vi "Parse Module Specifications.vi"(11 "Module Spec. File":path) -> (0 "Type Categories":T1, 1 "Namespaces":T12[](array[typedef]), 2 "Projections":T13[](array[typedef]), 3 "Module Name":string)   [LabVIEW 2013]
uses:
  Data Structures/JSON/Projection Info.ctl
  Data Structures/JSON/Namespace.ctl
  Data Structures/JSON/Enum.ctl
  Data Structures/JSON/Enum Value.ctl
  Data Structures/JSON/Method.ctl
  Data Structures/JSON/Param.ctl
  Data Structures/JSON/Connector Pane.ctl
  Data Structures/JSON/Connector Pane Terminal.ctl
  Data Structures/JSON/Type Categories.ctl
  Data Structures/JSON/TypeConv.ctl
  Data Structures/JSON/Simple Struct.ctl
  Data Structures/JSON/Class.ctl
  Data Structures/JSON/Property.ctl
  <vilib>/addons/JSON API/JSON Object/JSON Object.lvclass
  <vilib>/addons/JSON API/JSON Value/JSON Value.lvclass
  <vilib>/addons/JSON API/JSON Scalar/JSON Scalar.lvclass
  <vilib>/addons/JSON API/Variant JSON/Variant JSON.lvlib
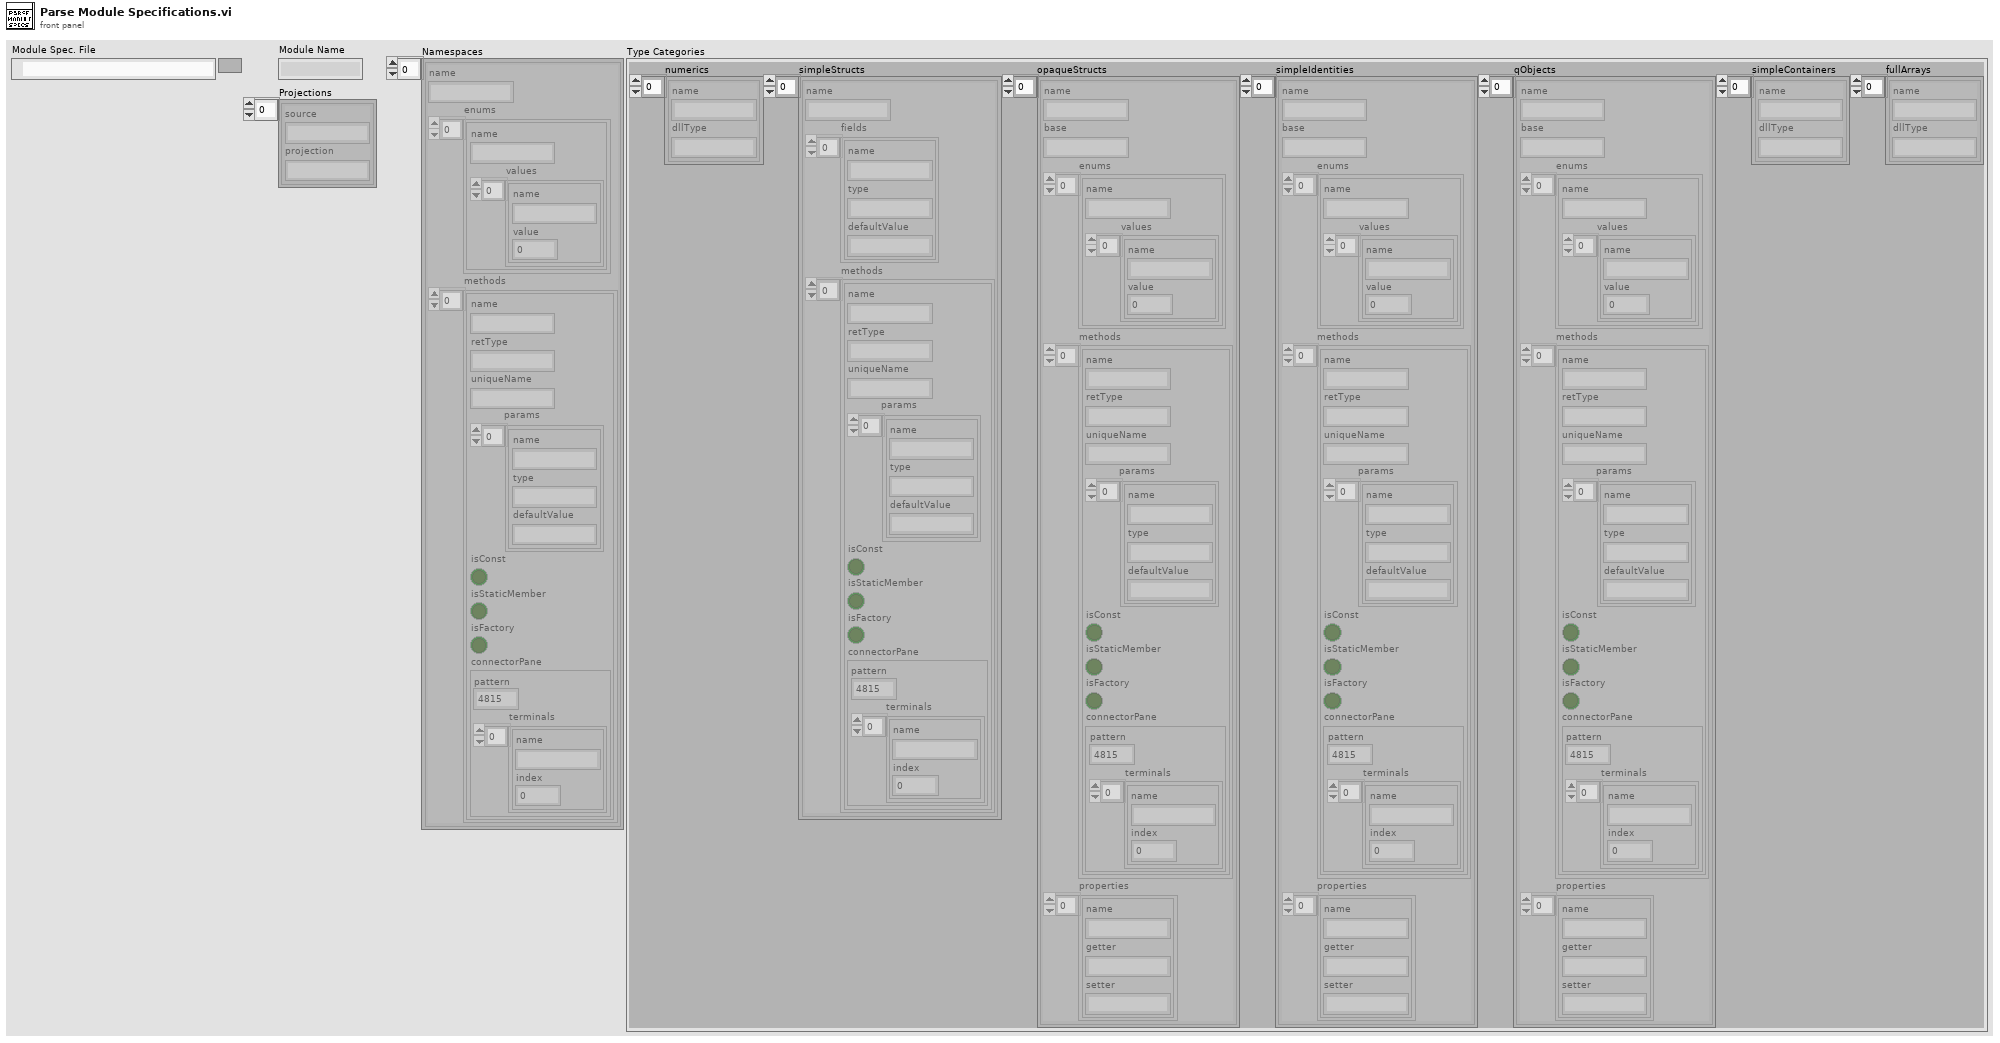
[diagram p1: front panel]
types:
  T1 = typedef "Type Categories.ctl" = cluster{"numerics":T2[], "simpleStructs":T3[], "opaqueStructs":T8[], "simpleIdentities":T8[], "qObjects":T8[], "simpleContainers":T2[], "fullArrays":T2[]}
  T2 = typedef "TypeConv.ctl" = cluster{"name":string, "dllType":string}
  T3 = typedef "Simple Struct.ctl" = cluster{"name":string, "fields":T4[], "methods":T5[]}
  T4 = typedef "Param.ctl" = cluster{"name":string, "type":string, "defaultValue":string}
  T5 = typedef "Method.ctl" = cluster{"name":string, "retType":string, "uniqueName":string, "params":T4[], "isConst":bool, "isStaticMember":bool, "isFactory":bool, "connectorPane":T6}
  T6 = typedef "Connector Pane.ctl" = cluster{"pattern":u32, "terminals":T7[]}
  T7 = typedef "Connector Pane Terminal.ctl" = cluster{"name":string, "index":u32}
  T8 = typedef "Class.ctl" = cluster{"name":string, "base":string, "enums":T9[], "methods":T5[], "properties":T11[]}
  T9 = typedef "Enum.ctl" = cluster{"name":string, "values":T10[]}
  T10 = typedef "Enum Value.ctl" = cluster{"name":string, "value":i32}
  T11 = typedef "Property.ctl" = cluster{"name":string, "getter":string, "setter":string}
  T12 = typedef "Namespace.ctl" = cluster{"name":string, "enums":T9[], "methods":T5[]}
  T13 = typedef "Projection Info.ctl" = cluster{"source":string, "projection":string}
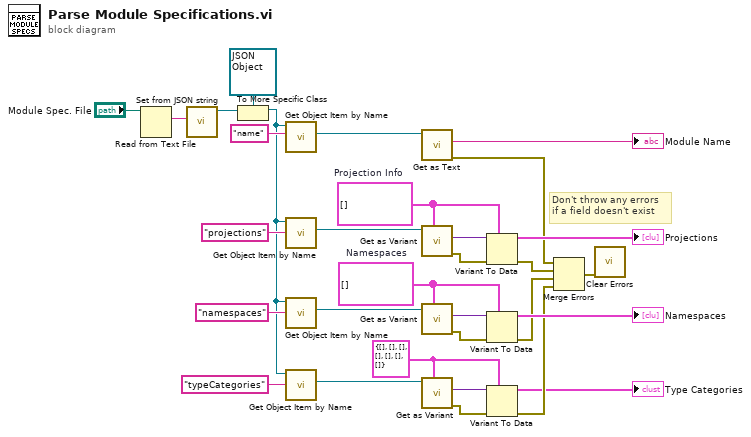
[diagram p0: block diagram]
diagram:
  w18 = T12[] []  # Namespaces
  w2 = T1 {"numerics"=[], "simpleStructs"=[], "opaqueStructs"=[], "simpleIdentities"=[], "qObjects"=[], "simpleContainers"=[], "fullArrays"=[]} ("Type Categories")
  w21 = T13[] []  # Projection Info
  # "Don't throw any errors\nif a field doesn't exist"
  n1 = Read from Text File(file (use dialog)="Module Spec. File") -> (text=w7:string)  [unwired: 3 in, 3 out]
  n2 = call <vilib>:"Set from JSON string.vi"("JSON stream"=w7) -> ("JSON Value out"=w29:refnum<class "JSON Value.lvclass">)  [unwired: 8 in, 2 out]
  n3 = To More Specific Class(target class=refnum<class "JSON Object.lvclass"> refnum ("JSON Object in"), reference=w29) -> (specific class reference=w24:refnum<class "JSON Object.lvclass">)  [unwired: 1 in, 1 out]
  n4 = call <vilib>:"Get Object Item by Name.vi"("name"="name", "JSON Value In"=w24) -> ("Value"=w23:refnum<class "JSON Value.lvclass">)  [unwired: 6 in, 3 out]
  n5 = call <vilib>:"Get Object Item by Name.vi"("name"="projections", "JSON Value In"=w24) -> ("Value"=w22:refnum<class "JSON Value.lvclass">)  [unwired: 6 in, 3 out]
  n6 = call <vilib>:"Get Object Item by Name.vi"("name"="namespaces", "JSON Value In"=w24) -> ("Value"=w17:refnum<class "JSON Value.lvclass">)  [unwired: 6 in, 3 out]
  n7 = call <vilib>:"Get Object Item by Name.vi"("name"="typeCategories", "JSON Value In"=w24) -> ("Value"=w4:refnum<class "JSON Value.lvclass">)  [unwired: 6 in, 3 out]
  n8 = call <vilib>:"Get as Text.vi"("JSON Scalar in"=w23) -> ("error out"=w11:errorcluster, "LabVIEW Text"=→"Module Name":string)  [unwired: 8 in, 1 out]
  n9 = call <vilib>:"Get as Variant.vi"("Variant (Data Type)"=w21, "JSON Scalar in"=w22) -> ("error out"=w13:errorcluster, "Variant out"=w20:variant)  [unwired: 7 in, 1 out]
  n10 = call <vilib>:"Get as Variant.vi"("Variant (Data Type)"=w18, "JSON Scalar in"=w17) -> ("error out"=w12:errorcluster, "Variant out"=w19:variant)  [unwired: 7 in, 1 out]
  n11 = call <vilib>:"Get as Variant.vi"("Variant (Data Type)"=w2, "JSON Scalar in"=w4) -> ("error out"=w6:errorcluster, "Variant out"=w5:variant)  [unwired: 7 in, 1 out]
  n12 = Variant To Data(error in=w13, type=w21, Variant=w20) -> (data=→"Projections":T13[], error out=w10:errorcluster)
  n13 = Variant To Data(error in=w12, type=w18, Variant=w19) -> (data=→"Namespaces":T12[], error out=w9:errorcluster)
  n14 = Variant To Data(error in=w6, type=w2, Variant=w5) -> (data=→"Type Categories":T1, error out=w3:errorcluster)
  n15 = Merge Errors(w11, w10, w9, w3) -> (w8:errorcluster)
  n16 = call <vilib>:"Clear Errors.vi"("error in (no error)"=w8) -> ()  [unwired: 6 in, 1 out]
